vi "Replace_Displacement_in_Columns-2.vi"(3 "[IN] Value for replace":dbl, 4 "[IN] Index of Displ":i32, 5 "[IN] Replaced Array":dbl[](array[numeric])) -> (2 "[OUT] Replaced Array":dbl[](array[numeric]))   [LabVIEW 2017]
doc: "Labelling of displacement for further deleting"
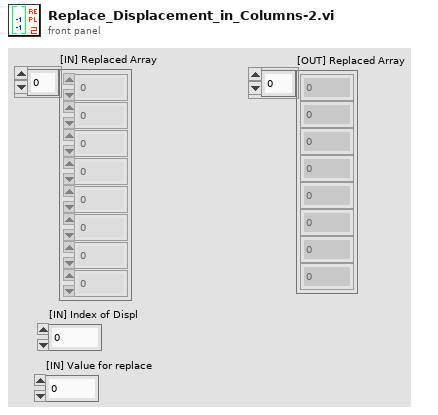
[diagram p1: front panel]
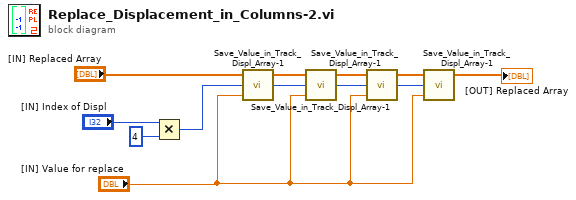
[diagram p0: block diagram]
diagram:
  n1 = Multiply(x="[IN] Index of Displ", y=4) -> (x*y=w9:i32)
  n2 = call "Save_Value_in_Track_Displ_Array-1.vi"("[IN] Value"="[IN] Value for replace", "[IN] Index"=w9, "[IN] Empty tracks\nfor points saving"="[IN] Replaced Array") -> ("[OUT] Index ++"=w7:i32, "[OUT Track with saved value"=w8:dbl[])  [unwired: 1 in]
  n3 = call "Save_Value_in_Track_Displ_Array-1.vi"("[IN] Value"="[IN] Value for replace", "[IN] Index"=w7, "[IN] Empty tracks\nfor points saving"=w8) -> ("[OUT] Index ++"=w5:i32, "[OUT Track with saved value"=w6:dbl[])  [unwired: 1 in]
  n4 = call "Save_Value_in_Track_Displ_Array-1.vi"("[IN] Value"="[IN] Value for replace", "[IN] Index"=w5, "[IN] Empty tracks\nfor points saving"=w6) -> ("[OUT] Index ++"=w3:i32, "[OUT Track with saved value"=w4:dbl[])  [unwired: 1 in]
  n5 = call "Save_Value_in_Track_Displ_Array-1.vi"("[IN] Value"="[IN] Value for replace", "[IN] Index"=w3, "[IN] Empty tracks\nfor points saving"=w4) -> ("[OUT Track with saved value"=→"[OUT] Replaced Array":dbl[])  [unwired: 1 in, 1 out]
